vi "swerve_globals.vi"() -> ()   [LabVIEW 2020]
panel:
  in  "Field Oriented?":bool
  out "Swerve Rotate Command":dbl
  out "Swerve Forwards Command":dbl
  out "Swerve Strafe Command":dbl
  out "Delta Theta (deg)":dbl
  out "Robot Position X (in)":dbl
  out "Robot Position Y (in)":dbl
  out "Gyro Theta (deg)":dbl
  out "Gyro Raw (deg)":dbl
  out "EncoderBR":dbl
  out "Encoder BL":dbl
  out "Encoder FL":dbl
  out "Encoder FR":dbl
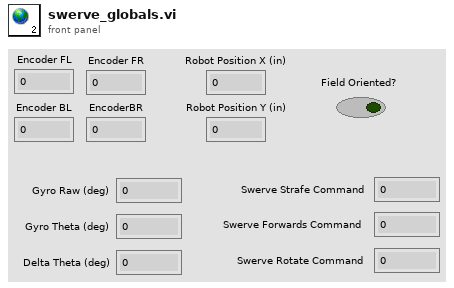
[diagram p1: front panel]
diagram:
